vi "Grab and Select Video Mode.vi"() -> ()   [LabVIEW 2018]
doc: "The Grab and Select Mode VI acquires images continuously and displays the images in an image control using high-level acquisition VIs. This example also demonstrates the capability to enumerate and change the video mode. A grab is appropriate for high-speed applications in which you need to process only one image at a time. This example requires a FireWire camera."
uses:
  <vilib>/vision/driver/NI_Vision_Acquisition_Software.lvlib
  <resource>/objmgr/imaqdx.rc
panel:
  out "Frame Rate":dbl(knob) scale=0.0..100.0
  in  "Camera Name":refnum<k21> caption="IMAQdx Session"
  out "Buffer Number":u32
  out "Image":T1(plugin-control)
  in  "Stop":bool
  in  "Video Modes":i32(listbox)
  # "Overview: Demonstrates how to enumerate the available video modes for a firewire camera and dynamically change which video mode is used.\nRequirements: Vision Acquisition Software, a firewire camera\nInstructions:\n1. Select the Camera Name\n2. Run the VI\n3. Select an available Video Mode"
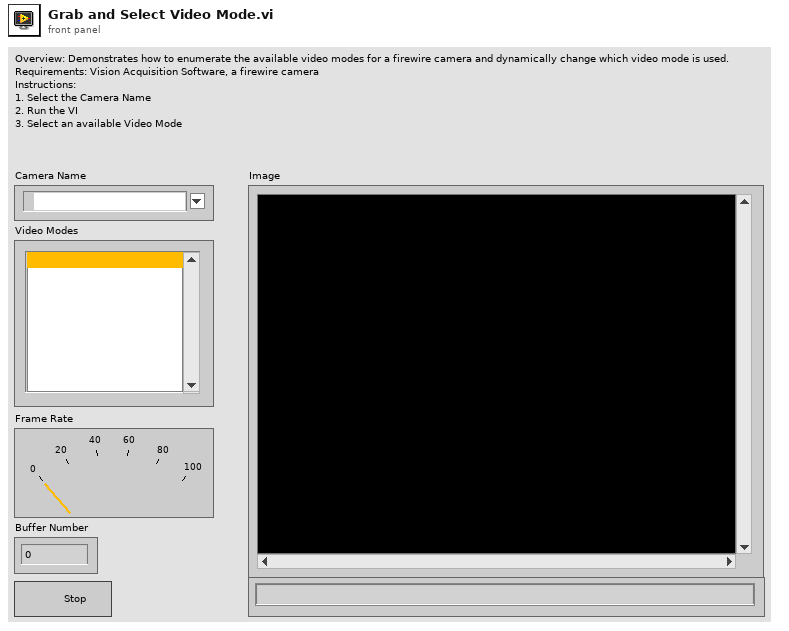
[diagram p1: front panel]
types:
  T1 = typedef "IMAQ Image.ctl" = refnum<image>
  T2 = typedef "IMAQdx.ctl" = refnum<k21>
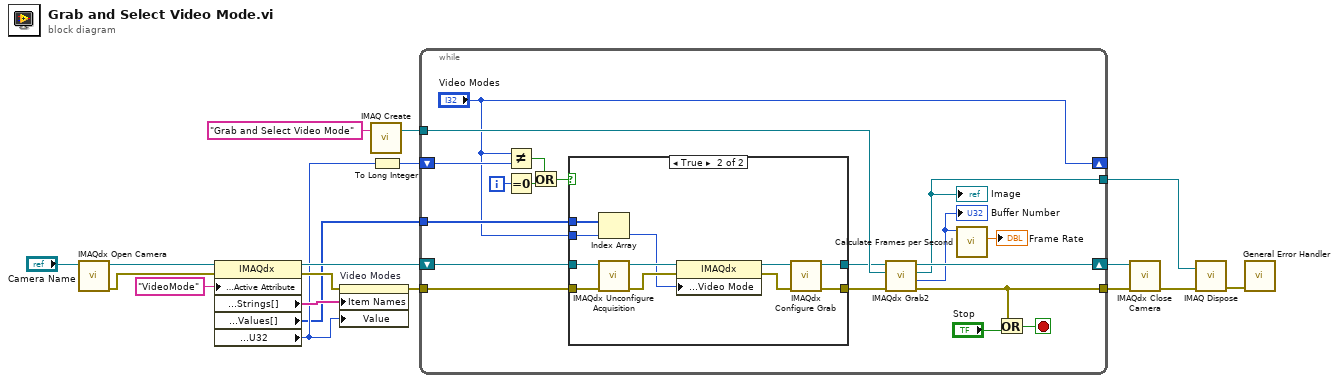
[diagram p0: block diagram]
diagram:
  n1 = call <vilib>:"IMAQdx Open Camera.vi"("Session In"="Camera Name") -> ("error out"=w11:errorcluster, "Session Out"=w13:T2)  [unwired: 2 in, 7 out]
  n2 = property class="IMAQdx"(reference=w13, error in=w11, "Camera Attributes:Active Attribute"="VideoMode" ("ActiveAttribute")) -> (reference out=w9:T2, error out=w10:errorcluster, "Camera Attributes:Enum:Strings[]"=w7:string[], "Camera Attributes:Enum:Values[]"=w1:u32[], "Camera Attributes:Value:U32"=w6:u32)
  n3 = property on="Video Modes" class="LstBox (strict)"(error in=w10, "Item Names"=w7, "Value"=w6) -> (error out=w8:errorcluster)  [unwired: 1 in, 1 out]
  n4 = call "IMAQ Create"("Image Name"="Grab and Select Video Mode") -> ("New Image"=w16:T1)  [unwired: 3 in, 2 out]
  n5 = To Long Integer(number=w6) -> (32bit integer=w5:i32)
  n6 = while {
    tunnel: w1 -> [w34]
    shift-left: w5 -> [w31]
    shift-right: ["Video Modes"] -> _
    tunnel: w16 -> [w35]
    tunnel: w8 -> [w36]
    tunnel: [w20] -> w18
    shift-right: [w23] -> w15
    shift-left: w9 -> [w37]
    tunnel: [w19] -> w4
    i -> [w27]
    stop <- w32 stop-if-true
    n7 = Not Equal?(x="Video Modes", y=w31) -> (x != y?=w28:bool)
    n8 = Equal To 0?(x=w27) -> (x = 0?=w26:bool)
    n9 = Or(x=w28, y=w26) -> (x .or. y?=w29:bool)
    n10 = case shown="True" w29 {
      tunnel: w37 -> [w39 w48]
      tunnel: w36 -> [w38 w47]
      tunnel: [w39 w44] -> w24
      tunnel: [w38 w45] -> w25
      tunnel: w34 -> [_ w50]
      tunnel: "Video Modes" -> [_ w49]
      frame False {
      }
      frame True {
        n11 = Index Array(array=w50, index=w49) -> (element=w40:u32)
        n12 = call <vilib>:"IMAQdx Unconfigure Acquisition.vi"("error in"=w47, "Session In"=w48) -> ("error out"=w41:errorcluster, "Session Out"=w46:T2)  [unwired: 8 out]
        n13 = property class="IMAQdx"(reference=w46, error in=w41, "Acquisition Attributes:Video Mode"=w40) -> (reference out=w43:T2, error out=w42:errorcluster)
        n14 = call <vilib>:"IMAQdx Configure Grab.vi"("error in"=w42, "Session In"=w43) -> ("error out"=w45:errorcluster, "Session Out"=w44:T2)  [unwired: 1 in, 7 out]
      }
    }
    n15 = call <vilib>:"IMAQdx Grab2.vi"("error in"=w25, "Image In"=w35, "Session In"=w24) -> ("error out"=w20:errorcluster, "Buffer Number Out"=w21:u32, "Image Out"=w19:T1, "Session Out"=w23:T2)  [unwired: 5 in]
    "Image" <- w19
    "Buffer Number" <- w21
    n16 = call <vilib>:"Calculate Frames per Second.vi"("Buffer Number"=w21) -> ("Processed Frames/s"=→"Frame Rate":dbl)  [unwired: 8 in, 2 out]
    n17 = Or(x=w20, y="Stop") -> (x .or. y?=w32:bool)
  }
  n18 = call <vilib>:"IMAQdx Close Camera.vi"("error in"=w18, "Session In"=w15) -> ("error out"=w3:errorcluster)  [unwired: 9 out]
  n19 = call "IMAQ Dispose"("Image"=w4, "error in (no error)"=w3) -> ("error out"=w2:errorcluster)  [unwired: 4 in]
  n20 = call <vilib>:"General Error Handler.vi"("error in (no error)"=w2) -> ()  [unwired: 2 in, 13 out]
